vi "LineStyle_Create.vi"(1 "lineStyle":T1 caption="stroke", 5 "error in (no error)":errorcluster) -> (14 "reference out":refnum<class "LineStyle.lvclass">, 19 "error out":errorcluster)   [LabVIEW 2014, in "LineStyle.lvclass"]
doc: "Creates and initializes a new LineStyle object.\n\nThis object should be destroyed using a LineStyle destructor VI.\n\n[GOOP 2.1]"
uses:
  <resource>/Framework/Providers/Open_GDS/UML/LineStyle_class/LineStyle.lvclass
  <resource>/Framework/Providers/Open_GDS/UML/LineStyle_class/LineStyleType.ctl
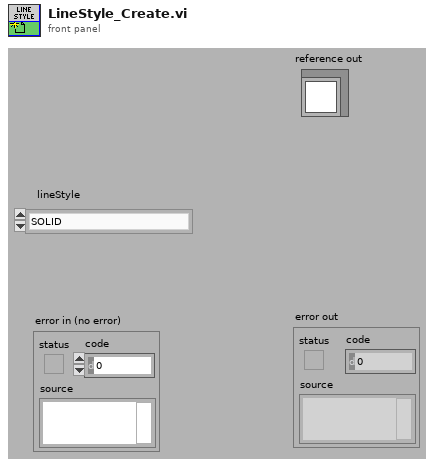
[diagram p1: front panel]
types:
  T1 = typedef "LineStyle.lvclass/LineStyleType.ctl" = enum16{"SOLID", "DOTTED"}
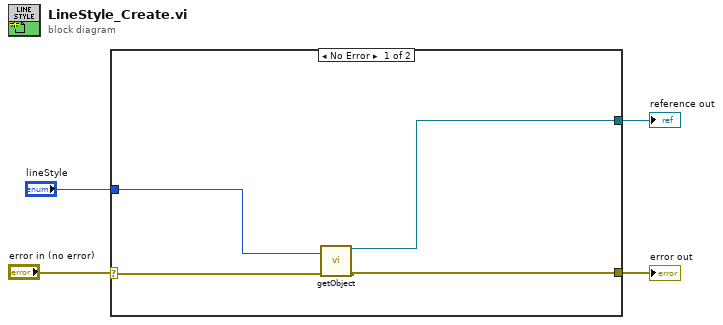
[diagram p0: block diagram]
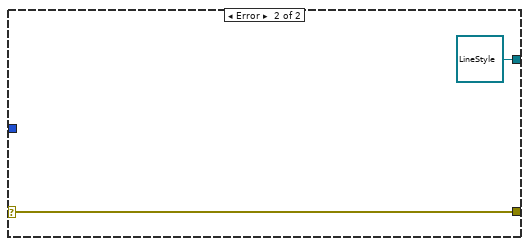
[diagram p2: hidden frame]
diagram:
  n1 = case shown="No Error" "error in (no error)" {
    selector: "error in (no error)" -> [w8 w10]
    tunnel: [w6 refnum<class "LineStyle.lvclass"> refnum ("reference out")] -> w4
    tunnel: [w7 w10] -> w3
    tunnel: "lineStyle" -> [w5 _]
    frame No Error {
      n2 = call <resource>:"getObject.vi"("lineStyle"=w5, "error in (no error)"=w8) -> ("reference out"=w6:refnum<class "LineStyle.lvclass">, "error out"=w7:errorcluster)  [unwired: 16 in]
    }
    frame Error {
    }
  }
  "error out" <- w3
  "reference out" <- w4
